vi "Max Read Array.vi"(8 "error in":errorcluster, 11 "Max Voltage Limit in":refnum<class "Voltage Limit.lvclass">) -> (0 "error out":errorcluster, 1 "Changed or First Call?":bool, 2 "Voltage Max SP":dbl[](array[numeric]), 3 "Max Voltage Limit out":refnum<class "Voltage Limit.lvclass">)   [LabVIEW 2023, in "Voltage Limit.lvclass"]
uses:
  Voltage Limit.lvclass
  Parents/Limit/Limit.lvclass
  Voltage Limit.lvclass/Voltage Limit.ctl
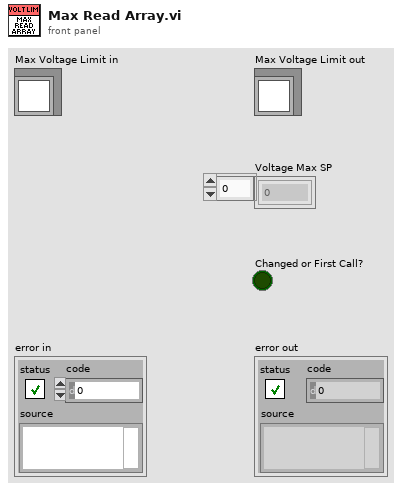
[diagram p1: front panel]
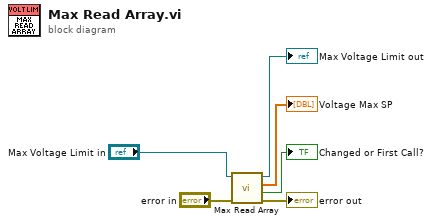
[diagram p0: block diagram]
diagram:
  n1 = call-parent "Max Read Array.vi"("error in"="error in", "Max Limit in"="Max Voltage Limit in") -> ("error out"=→"error out":errorcluster, "Changed or First Call?"=→"Changed or First Call?":bool, "Current Max Limit"=→"Voltage Max SP":dbl[], "Max Limit out"=→"Max Voltage Limit out":refnum<class "Voltage Limit.lvclass">)  [unwired: 6 in]
